vi "Close.vi"(8 "error in (no error)":errorcluster, 11 "HAL.Serial in":refnum<class "HAL.Serial.lvclass">) -> (0 "error out":errorcluster, 3 "HAL.Serial out":refnum<class "HAL.Serial.lvclass">)   [LabVIEW 2019, in "Instrument.lvlib" / "HAL.Serial.lvclass"]
uses:
  HAL.Serial.lvclass
  HAL.Serial.lvclass/HAL.Serial.ctl
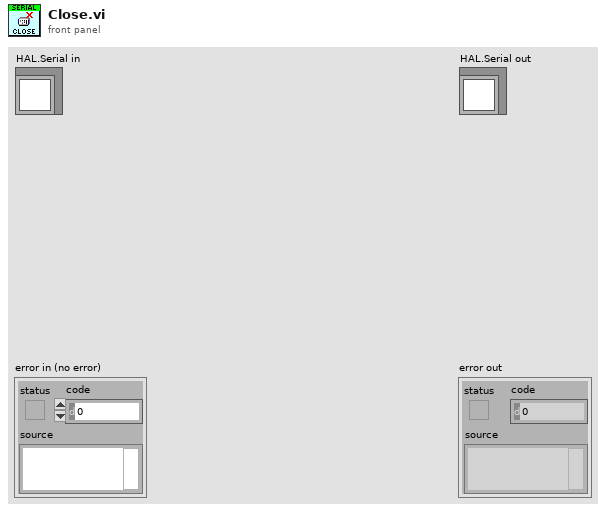
[diagram p1: front panel]
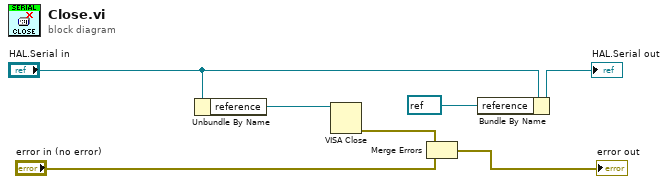
[diagram p0: block diagram]
diagram:
  n1 = Unbundle By Name("HAL.Serial in") -> ("reference"=w3:refnum<visa-resource-name>)
  n2 = VISA Close(VISA resource name=w3) -> (error out=w2:errorcluster)  [unwired: 1 in]
  n3 = Merge Errors(w2, "error in (no error)") -> (→"error out":errorcluster)
  n4 = Bundle By Name(cluster="HAL.Serial in", "reference"=refnum<visa-resource-name> refnum ("VISA resource name")) -> (→"HAL.Serial out":refnum<class "HAL.Serial.lvclass">)
